vi "Write Interface object handle.vi"(8 "error in (no error)":errorcluster, 10 "ObjHandle":T1, 11 "DeviceNET in":refnum<class "DeviceNET.lvclass">) -> (0 "error out":errorcluster, 3 "DeviceNET out":refnum<class "DeviceNET.lvclass">)   [LabVIEW 2016, in "DeviceNET.lvclass"]
uses:
  DeviceNET.lvclass
  <vilib>/DeviceNet/VIAPI/subVIs/xobjhandle.ctl
  DeviceNET.lvclass/DeviceNET.ctl
  <vilib>/DeviceNet/DeviceNetLIB.lvlib
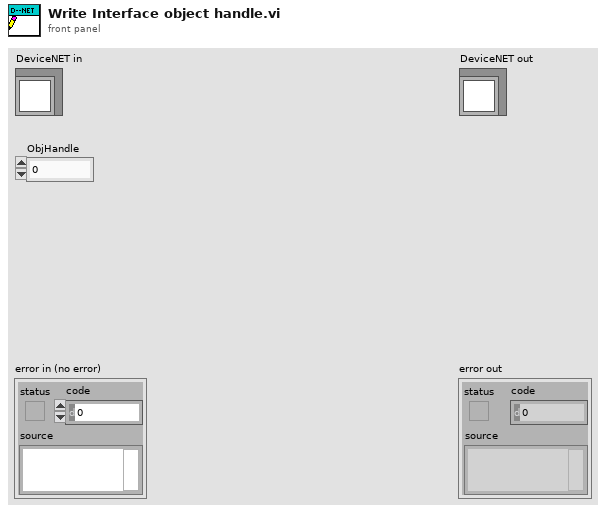
[diagram p1: front panel]
types:
  T1 = typedef "DeviceNetLIB.lvlib/xobjhandle.ctl" = u32
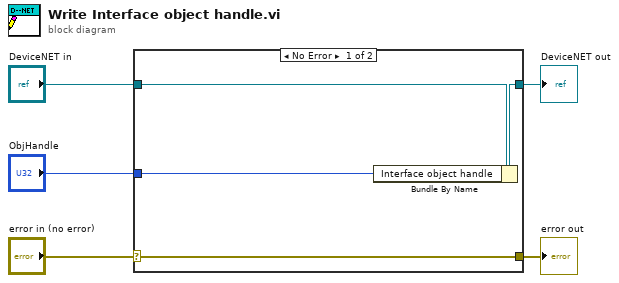
[diagram p0: block diagram]
diagram:
  n1 = case shown="No Error" "error in (no error)" {
    selector: "error in (no error)" -> [w9 w10]
    tunnel: [w9 w10] -> w4
    tunnel: [w7 w11] -> w2
    tunnel: "DeviceNET in" -> [w8 w11]
    tunnel: "ObjHandle" -> [w6 _]
    frame No Error {
      n2 = Bundle By Name(cluster=w8, "Interface object handle"=w6) -> (w7:refnum<class "DeviceNET.lvclass">)
    }
    frame Error {
    }
  }
  "error out" <- w4
  "DeviceNET out" <- w2
